vi "NewPort_PM_USB_Read-Set.vi"(0 "Dual: CH_1 \nLambda (nm)":i32, 1 "reference":refnum<k24>, 2 "USB Address":i32, 3 "Read Power(F)\nSet Lambda(T)":bool, 5 "Dual: CH_2 \nLambda (nm)":i32, 9 "Single: CH\nLambda (nm)":i32, 11 "error in":errorcluster, 12 "Pick Single CH \nCH1(F)\nCH2(T)":bool, 13 "Set Lambda\nSingle CH(F)\nDual CHs(T)":bool, 14 "Read Power\nSingle CH(F)\nDual CHs(T)":bool) -> (4 "Query-String Format\nfrom Read Buffer":string, 15 "error out":errorcluster)   [LabVIEW 2017]
uses:
  C:/Program Files (x86)/Newport/Newport USB Driver/Bin/UsbDllWrap.dll
  Program Files (x86)/Newport/Newport USB Driver/Bin/UsbDllWrap.dll
panel:
  out "Query-Double Format\nfrom Read Buffer":dbl
  # "This VI switches between set command and query command to the Newport power meter\nand returns query values/info in string format."
  # "Outputs"
  # "Inputs"
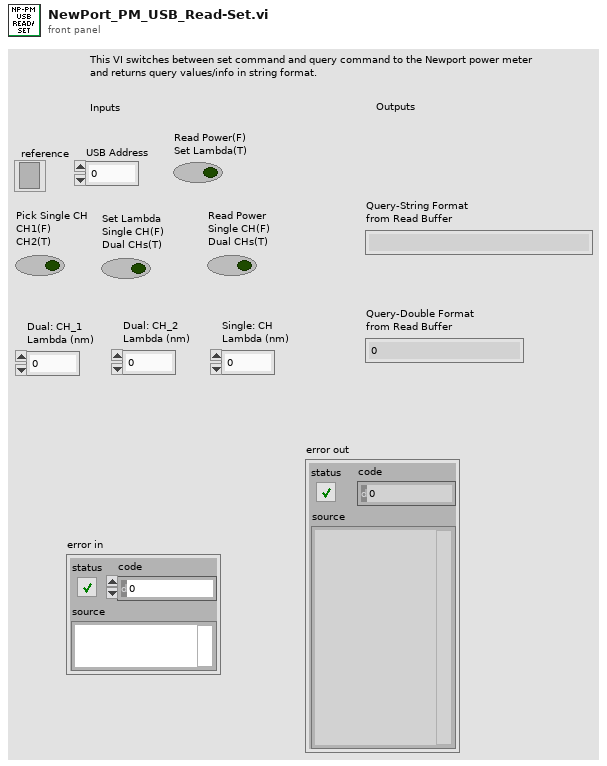
[diagram p1: front panel]
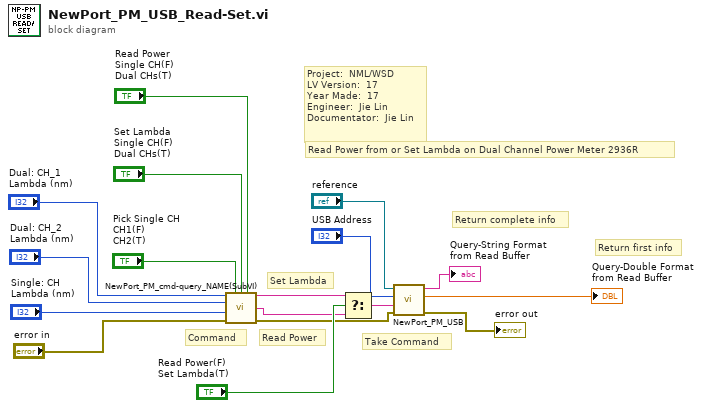
[diagram p0: block diagram]
diagram:
  # "Project:  NML/WSD \nLV Version:  17\nYear Made:  17\nEngineer:  Jie Lin\nDocumentator:  Jie Lin"
  # "Take Command"
  # "Command"
  # "Return first info"
  # "Return complete info"
  # "Set Lambda"
  # "Read Power"
  # "Read Power from or Set Lambda on Dual Channel Power Meter 2936R"
  n1 = call "NewPort_PM_cmd-query_NAME(SubVI).vi"("Dual: CH_1 \nLambda (nm)"="Dual: CH_1 \nLambda (nm)", "Pick Single CH \nCH1(F)\nCH2(T)"="Pick Single CH \nCH1(F)\nCH2(T)", "Set Lambda\nSingle CH(F)\nDual CHs(T)"="Set Lambda\nSingle CH(F)\nDual CHs(T)", "Read Power\nSingle CH(F)\nDual CHs(T)"="Read Power\nSingle CH(F)\nDual CHs(T)", "Dual: CH_2\nLambda (nm)"="Dual: CH_2 \nLambda (nm)", "Single: CH\nLambda (nm)"="Single: CH\nLambda (nm)", "error in (no error)"="error in") -> ("Set Lambda (nm)"=w4:string, "Read Power (W)"=w5:string, "error out"=w8:errorcluster)  [unwired: 6 in]
  n2 = Select(t=w4, s="Read Power(F)\nSet Lambda(T)", f=w5) -> (s? t:f=w16:string)
  n3 = call "NewPort_PM_USB.vi"("error in"=w8, "PM:CMD_QUERY In"=w16, "USB Address"="USB Address", "reference"="reference") -> ("error out"=→"error out":errorcluster, "Query-Double\nfrom Read Buffer\nFirst Info"=→"Query-Double Format\nfrom Read Buffer":dbl, "Query-String\nfrom Read Buffer\nComplete Info"=→"Query-String Format\nfrom Read Buffer":string)  [unwired: 5 in]
